vi "Stitching-Core.vi"(5 "selected rows":i32[](array[numeric]), 6 "column":i32, 8 "error in (no error)":errorcluster, 9 "Z-planes":i32, 10 "Item Names":string[][](array[string]), 11 "Base directory containing all dataset folders":path) -> (0 "error out":errorcluster)   [LabVIEW 2013]
uses:
  Coordinates list window/Globals/Coord window-Globals.vi
  <vilib>/vision/NI_Vision_Development_Module.lvlib
panel:
  out "appended path":path
  out "Z-plane":i32
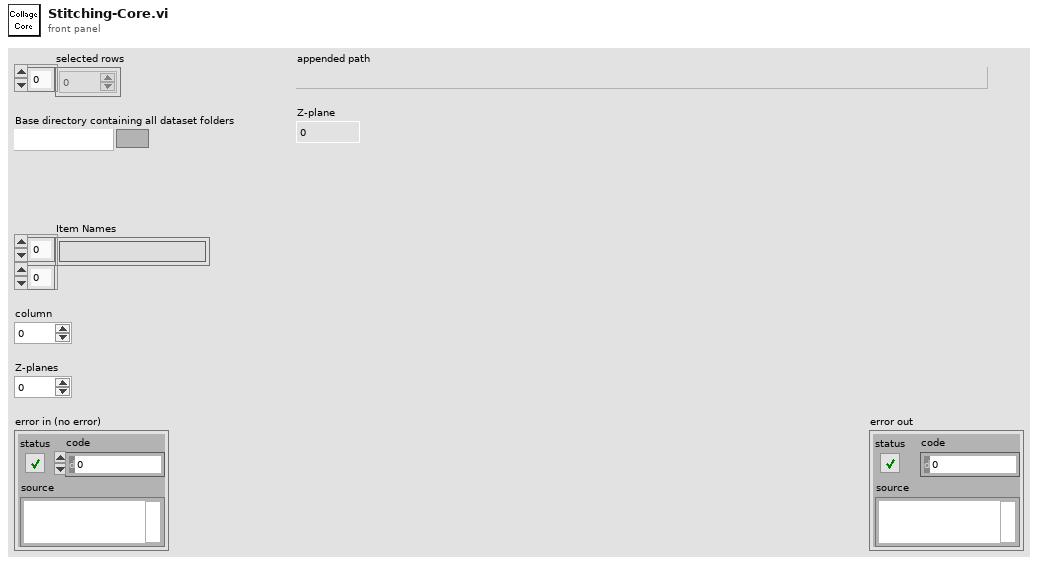
[diagram p1: front panel]
types:
  T1 = typedef "IMAQ Image.ctl" = refnum<image>
  T2 = cluster{"X min (um) ":i32, "Y min (um)":i32, "Size reduction multiplier":dbl}
  T3 = typedef "Image Type" = u32
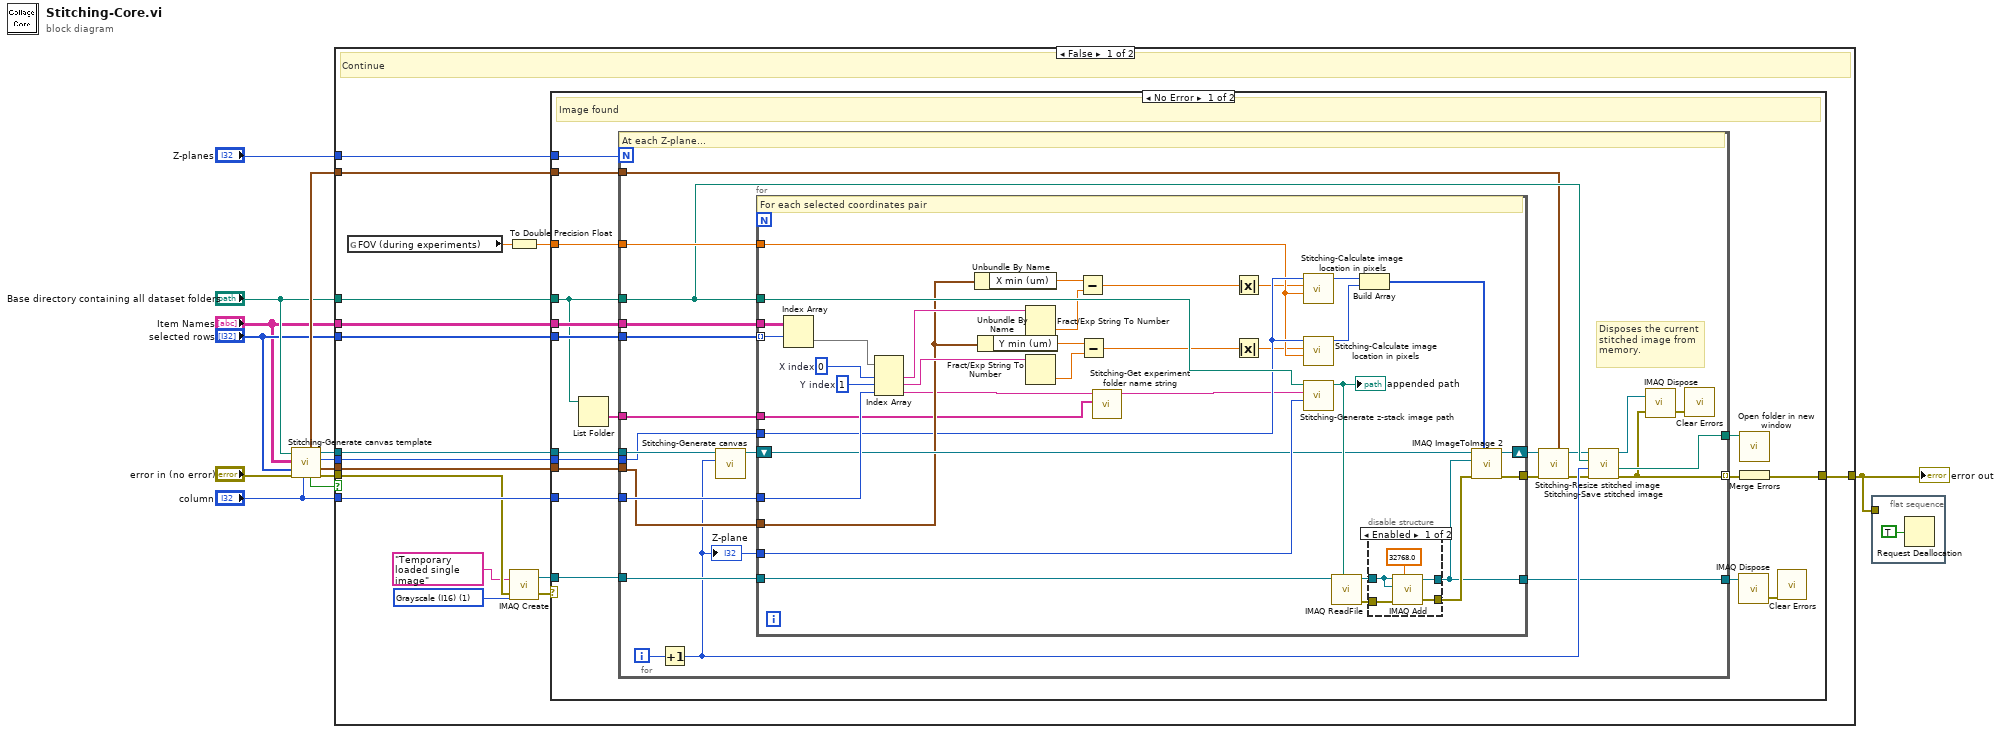
[diagram p0: block diagram]
diagram:
  n1 = call "Stitching-Generate canvas template.vi"("Experiment folder names column to use"="column", "error in (no error)"="error in (no error)", "Selected rows"="selected rows", "Item Names"="Item Names", "Base directory containing all dataset folders"="Base directory containing all dataset folders") -> ("error out"=w9:errorcluster, "Min"=w6:cluster{"X min (um) ":dbl, "Y min (um)":dbl}, "Single image size (pixels)"=w7:i32, "Canvas"=w5:T1, "Cancelled?"=w13:bool, "Stitched image setup"=w12:T2)  [unwired: 1 in]
  n2 = case shown="False" w13 {
    tunnel: "column" -> [w30 _]
    tunnel: "Z-planes" -> [w29 _]
    tunnel: w5 -> [w27 _]
    tunnel: w6 -> [w26 _]
    tunnel: w7 -> [w25 _]
    tunnel: "Item Names" -> [w24 _]
    tunnel: w9 -> [w23 _]
    tunnel: [w20 _] -> w1
    tunnel: "selected rows" -> [w19 _]
    tunnel: "Base directory containing all dataset folders" -> [w18 _]
    tunnel: w12 -> [w17 _]
    frame False {
      w22 = T3 1 items=["Grayscale (U8)", "Grayscale (I16)", "Grayscale (SGL)", "Complex (CSG)", "RGB (U32)", "HSL (U32)", "RGB (U64)", "Grayscale (U16)"] ("Image Type")
      # "Continue"
      n3 = global read "Coord window-Globals.vi" "FOV (during experiments)"() -> (w15:sgl)
      n4 = call "IMAQ Create"("Image Name"="Temporary loaded single image", "Image Type"=w22, "error in (no error)"=w23) -> ("New Image"=w28:T1, "error out"=w21:errorcluster)  [unwired: 2 in]
      n5 = To Double Precision Float(number=w15) -> (double precision float=w14:dbl)
      n6 = case shown="No Error" w21 {
        selector: w21 -> [_ w114]
        tunnel: w19 -> [w47 _]
        tunnel: w30 -> [w46 _]
        tunnel: w18 -> [w34 _]
        tunnel: w29 -> [w45 _]
        tunnel: w28 -> [w44 _]
        tunnel: w27 -> [w43 _]
        tunnel: w26 -> [w42 _]
        tunnel: w25 -> [w41 _]
        tunnel: w14 -> [w40 _]
        tunnel: w24 -> [w39 _]
        tunnel: [w36 w114] -> w20
        tunnel: w17 -> [w31 _]
        frame No Error {
          # "Image found"
          n7 = List Folder(path=w34) -> (folder names=w33:string[])  [unwired: 3 in, 3 out]
          n8 = for {
            N: w45 -> [_]
            tunnel: w47 -> [w67]
            tunnel: w39 -> [w68]
            tunnel: w46 -> [w70]
            tunnel: w34 -> [w60]
            tunnel: w44 -> [w69]
            tunnel: w43 -> [w65]
            tunnel: w42 -> [w63]
            tunnel: w41 -> [w62]
            tunnel: w40 -> [w61]
            tunnel: [w58] -> w38
            tunnel: [w54] -> w37 mode=indexing
            tunnel: w33 -> [w57]
            tunnel: [w56] -> w32
            tunnel: w31 -> [w48]
            i -> [w66]
            # "Disposes the current stitched image from memory."
            # "At each Z-plane..."
            n9 = Increment(x=w66) -> (x+1=w59:i32)
            "Z-plane" <- w59
            n10 = call "Stitching-Generate canvas.vi"("File increment number / Z-plane number"=w59, "Canvas template"=w65) -> ("Stitched image"=w64:T1)  [unwired: 9 in]
            n11 = for {
              tunnel: w67 -> [w104] mode=indexing
              tunnel: w68 -> [w105]
              tunnel: w70 -> [w100]
              tunnel: w60 -> [w106]
              tunnel: w59 -> [w94]
              tunnel: w69 -> [w95]
              shift-right: [w80] -> w52
              shift-left: w64 -> [w93]
              tunnel: w63 -> [w90]
              tunnel: w62 -> [w85]
              tunnel: w61 -> [w84]
              tunnel: [w75] -> w50
              tunnel: [w74] -> w58
              tunnel: w57 -> [w73]
              w101 = 1  # Y index
              w102 = 0  # X index
              # "For each selected coordinates pair"
              n12 = Index Array(array=w105, index (row)=w104) -> (element=w103:string[])  [unwired: 1 in]
              n13 = Index Array(array=w103, index #1=w102, index #2=w101, index #3=w100) -> (element #1=w99:string, element #2=w98:string, element #3=w72:string)
              n14 = Unbundle By Name(w90) -> ("X min (um)"=w92:dbl)
              n15 = Unbundle By Name(w90) -> ("Y min (um)"=w89:dbl)
              n16 = Fract/Exp String To Number(string=w99) -> (number=w91:dbl)  [unwired: 3 in, 1 out]
              n17 = Fract/Exp String To Number(string=w98) -> (number=w88:dbl)  [unwired: 3 in, 1 out]
              n18 = Subtract(x=w92, y=w91) -> (x-y=w87:dbl)
              n19 = Subtract(x=w89, y=w88) -> (x-y=w86:dbl)
              n20 = call "Stitching-Get experiment folder name string.vi"("folder names"=w73, "Experiment folder user string"=w72) -> ("Actual experiment folder name"=w71:string)  [unwired: 9 in]
              n21 = Absolute Value(x=w87) -> (abs(x)=w79:dbl)
              n22 = Absolute Value(x=w86) -> (abs(x)=w78:dbl)
              n23 = call "Stitching-Calculate image location in pixels.vi"("FOV (um)"=w84, "Image location (um)"=w79, "Single image size (pixels)"=w85) -> ("image location within canvas (pixels)"=w83:i32)  [unwired: 8 in]
              n24 = call "Stitching-Calculate image location in pixels.vi"("FOV (um)"=w84, "Image location (um)"=w78, "Single image size (pixels)"=w85) -> ("image location within canvas (pixels)"=w82:i32)  [unwired: 8 in]
              n25 = call "Stitching-Generate z-stack image path.vi"("File increment number / Z-plane number"=w94, "Experiment folder name"=w71, "Base directory"=w106) -> ("appended path"=w96:path)  [unwired: 8 in]
              "appended path" <- w96
              n26 = call "IMAQ ReadFile"("File Path"=w96, "Image"=w95) -> ("error out"=w97:errorcluster, "Image Out"=w77:T1)  [unwired: 5 in, 3 out]
              n27 = Build Array(w83, w82) -> (w81:i32[])
              n28 = disable-structure shown="Enabled" {
                disable-tunnel: w97 -> [w110 w112]
                disable-tunnel: w77 -> [w109 w113]
                disable-tunnel: [w108 w112] -> w76
                disable-tunnel: [w107 w113] -> w74
                frame Enabled {
                  n29 = call "IMAQ Add"("Image Src A"=w109, "Constant"=32768.0, "Image Dst"=w109, "error in (no error)"=w110) -> ("Image Dst Out"=w107:T1, "error out"=w108:errorcluster)  [unwired: 3 in]
                }
                frame Disabled {
                }
              }
              n30 = call "IMAQ ImageToImage 2"("Offset Left/Top"=w81, "error in (no error)"=w76, "Image Src (Small)"=w74, "Image Src (Large)"=w93) -> ("error out"=w75:errorcluster, "Image Dst Out"=w80:T1)  [unwired: 2 in, 4 out]
            }
            n31 = call "Stitching-Resize stitched image.vi"("Stitched image setup"=w48, "error in (no error)"=w50, "Stitched image ref in"=w52) -> ("error out"=w51:errorcluster, "Stitched image ref"=w49:T1)  [unwired: 7 in]
            n32 = call "Stitching-Save stitched image.vi"("error in (no error)"=w51, "Z-plane"=w59, "Base directory containing all dataset folders"=w60, "Stitched image ref in"=w49) -> ("error out"=w54:errorcluster, "Collage folder"=w56:path, "Stitched image ref"=w55:T1)  [unwired: 5 in]
            n33 = call "IMAQ Dispose"("Image"=w55, "error in (no error)"=w54) -> ("error out"=w53:errorcluster)  [unwired: 4 in]
            n34 = call <vilib>:"Clear Errors.vi"("error in (no error)"=w53) -> ()  [unwired: 6 in, 1 out]
          }
          n35 = call "IMAQ Dispose"("Image"=w38) -> ("error out"=w35:errorcluster)  [unwired: 5 in]
          n36 = call "Open folder in new window.vi"("Directory to open"=w32) -> ()  [unwired: 10 in, 1 out]
          n37 = Merge Errors(w37) -> (w36:errorcluster)
          n38 = call <vilib>:"Clear Errors.vi"("error in (no error)"=w35) -> ()  [unwired: 6 in, 1 out]
        }
        frame Error {
        }
      }
    }
    frame True {
      # "Cancelled"
    }
  }
  "error out" <- w1
  n39 = flat-sequence {
    tunnel: w1 -> [_]
    frame #0 {
      n40 = Request Deallocation(TRUE ("flag")) -> ()
    }
  }
